vi "NI VeriStand - Generate PCI FPGA Clock.vi"(9 "Use External Timing":bool, 10 "Write to  RTSI":bool, 11 "Loop Rate (usec)":u32) -> ()   [LabVIEW 2010, in "NI_VS FPGA Clock Support.lvlib"]
uses:
  <userlib>/_NI VeriStand FPGA Support/NI VeriStand FPGA Clock Support/NI_VS FPGA Clock Support.lvlib
  <vilib>/eio/EIONode/EIONode.xnode
  <vilib>/rvi/eio/nirviEIOImplementation/nirviEIOImplementation.xnode
  <vilib>/rvi/eio/common/nirviEmuClasses.ctl
  <vilib>/eio/EIOMethodNode/EIOMethodNode.xnode
  <vilib>/rvi/eio/nirviEIOMethodImplementation/nirviEIOMethodImplementation.xnode
  <userlib>/_NI VeriStand FPGA Support/NI VeriStand FPGA Clock Support/NI VeriStand - Timing Engine Globals.vi
  <vilib>/rvi/eio/common/nirviEmuTemplateMethod_noerrors.vi
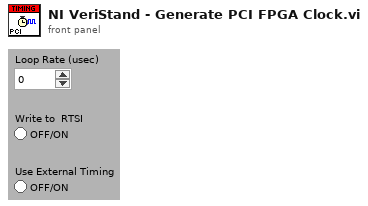
[diagram p1: front panel]
types:
  T1 = typedef "nirviEmuClasses.ctl" = enum16{"IO Read", "IO Write", "Method", "Property Read", "Property Write"}
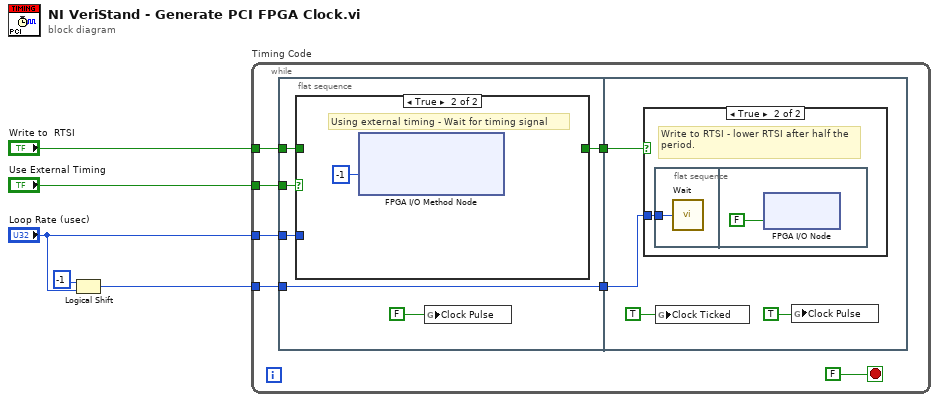
[diagram p0: block diagram]
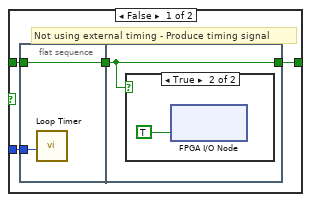
[diagram p2: hidden frame]
diagram:
  n1 = Logical Shift(y=i8 -1, x="Loop Rate (usec)") -> (x << y=w2:u32)
  n2 = while "Timing Code" {
    tunnel: w2 -> [w12]
    tunnel: "Loop Rate (usec)" -> [w11]
    tunnel: "Use External Timing" -> [w10]
    tunnel: "Write to  RTSI" -> [w9]
    stop <- FALSE stop-if-true
    n3 = flat-sequence {
      tunnel: w12 -> [w15]
      tunnel: w11 -> [w18]
      tunnel: w10 -> [w17]
      tunnel: w9 -> [w16]
      tunnel: [w15] -> w7
      tunnel: [w14] -> w6
      tunnel: w7 -> [w65]
      tunnel: w6 -> [w64]
      frame #0 {
        n4 = case shown="True" w17 {
          tunnel: w18 -> [w22 _]
          tunnel: w16 -> [w20 _]
          tunnel: [w19 _] -> w14
          frame False {
            # "Not using external timing - Produce timing signal"
            n5 = flat-sequence {
              tunnel: [w23] -> w21
              tunnel: w22 -> [w24]
              tunnel: w20 -> [w23]
              tunnel: w21 -> [w25]
              tunnel: [w25] -> w19
              frame #0 {
                n6 = call "Loop Timer"("Count(uSec)"=w24) -> ()  [unwired: 1 out]
              }
              frame #1 {
                n7 = case shown="True" w25 {
                  frame False {
                  }
                  frame True {
                    n8 = xnode "FPGA I/O Node"("RTSI0"=TRUE ("TRIG0")) -> ()  [unwired: 1 in, 1 out]
                  }
                }
              }
            }
          }
          frame True {
            # "Using external timing - Wait for timing signal"
            n9 = xnode "FPGA I/O Method Node"("Timeout"=-1) -> ()  [unwired: 1 in, 2 out]
          }
        }
        n10 = global write "NI VeriStand - Timing Engine Globals.vi" "Clock Pulse"(FALSE ("Clock Ticked")) -> ()
      }
      frame #1 {
        n11 = case shown="True" w64 {
          tunnel: w65 -> [_ w66]
          frame False {
          }
          frame True {
            # "Write to RTSI - lower RTSI after half the period."
            n12 = flat-sequence {
              tunnel: w66 -> [w67]
              frame #0 {
                n13 = call "Wait"("Count(uSec)"=w67) -> ()  [unwired: 1 out]
              }
              frame #1 {
                n14 = xnode "FPGA I/O Node"("RTSI0"=FALSE ("TRIG0")) -> ()  [unwired: 1 in, 1 out]
              }
            }
          }
        }
        n15 = global write "NI VeriStand - Timing Engine Globals.vi" "Clock Ticked"(TRUE ("Clock Ticked")) -> ()
        n16 = global write "NI VeriStand - Timing Engine Globals.vi" "Clock Pulse"(TRUE ("Clock Ticked")) -> ()
      }
    }
  }
